vi "Tank Controll.vi"() -> ()   [LabVIEW 2016]
uses:
  <vilib>/addons/control/pid/pid.llb/PID (DBL).vi
  <vilib>/addons/control/pid/NI_PID_pid.lvlib
  <vilib>/measure/NI_MABase.lvlib
panel:
  out "String 2":string
  out "String":string
  in  "Cycle Stop":bool
  in  "Start":bool
  in  "Position 2":bool
  in  "Position 1":bool
  out "Conveyor":bool
  out "Drop 2":bool
  out "Drop 1":bool
  out "Fill Two":bool
  out "Fill One":bool
  in  "Tank Controll":bool
  in  "Setpoint  2":dbl
  in  "level 2":dbl(slide) scale=0.0..10.0
  out "Pump on":bool
  in  "Setpoint":dbl
  in  "stop":bool
  in  "level":dbl(slide) scale=0.0..10.0
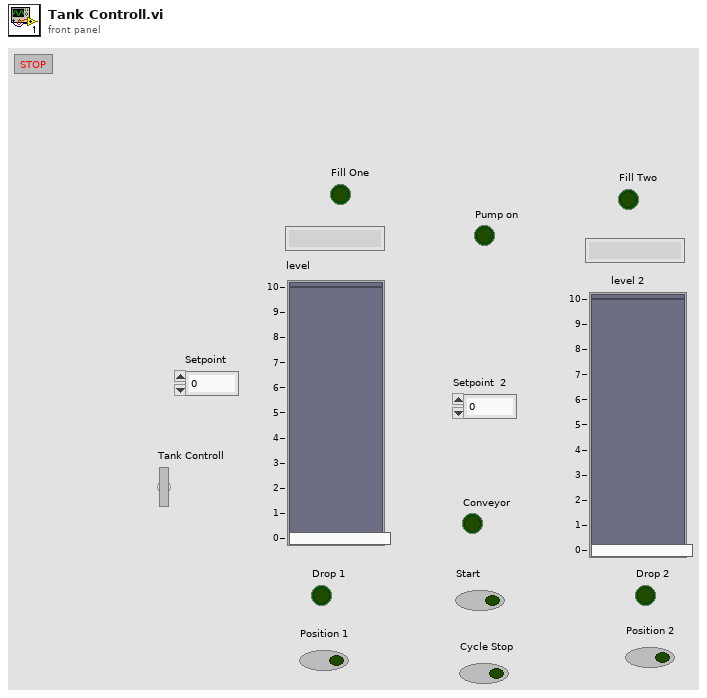
[diagram p1: front panel]
types:
  T1 = enum16{"Wait For Start", "Move Tank 1", "Fill One", "Move Tank 2", "Fill Two", "Move to Stop", "Stop All"}
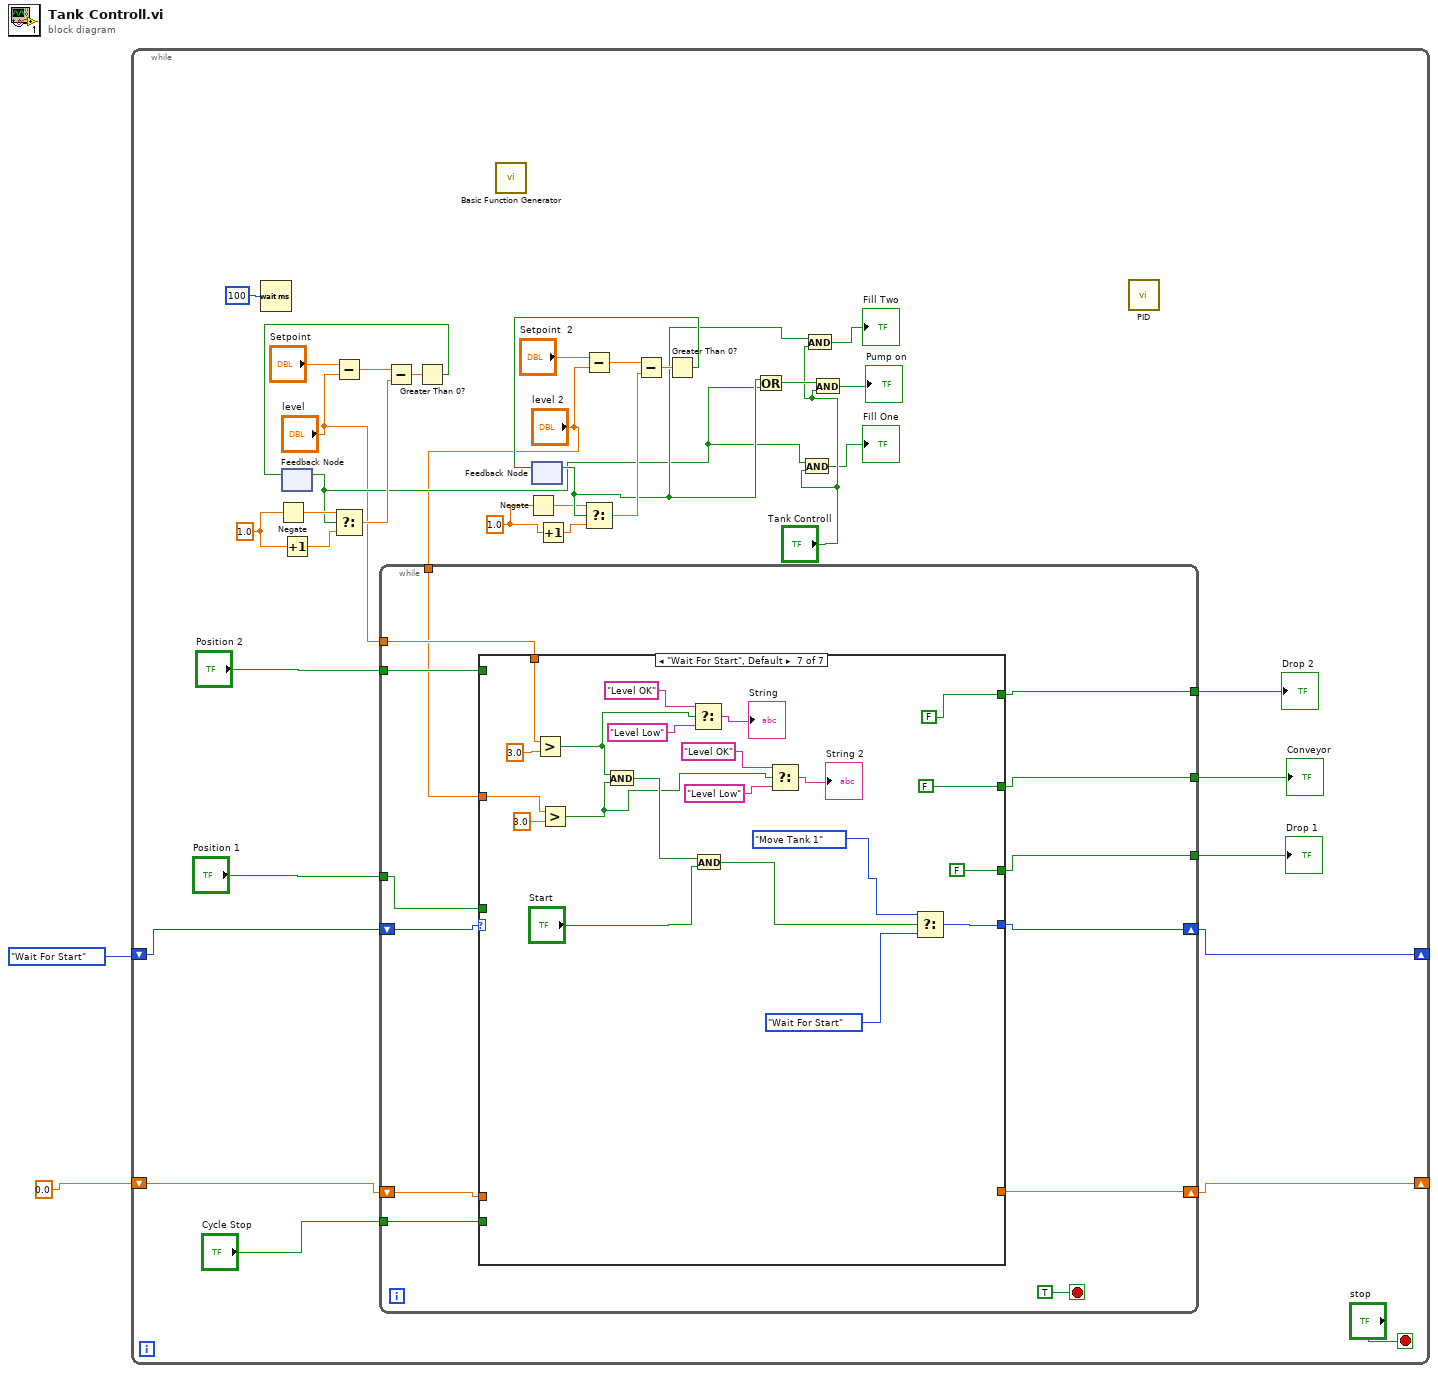
[diagram p0: block diagram]
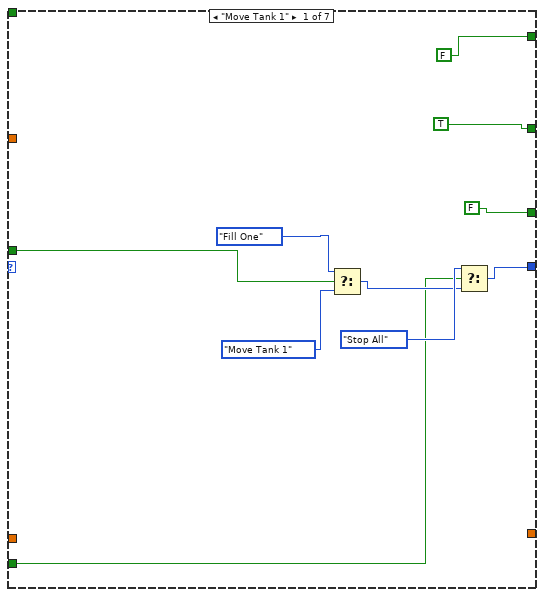
[diagram p2: hidden frame]
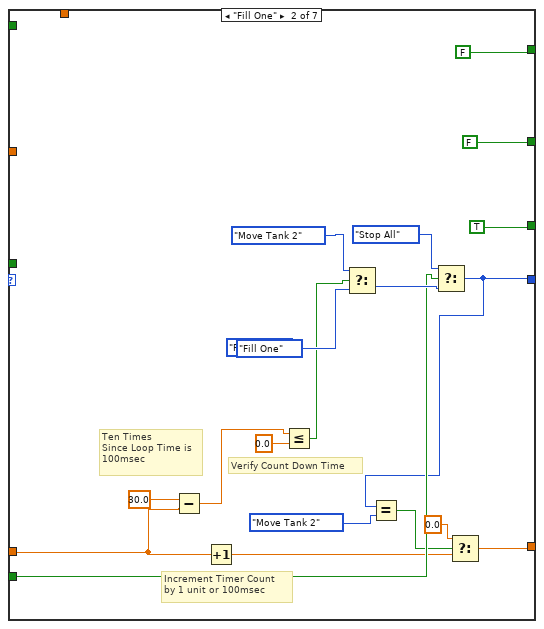
[diagram p3: hidden frame]
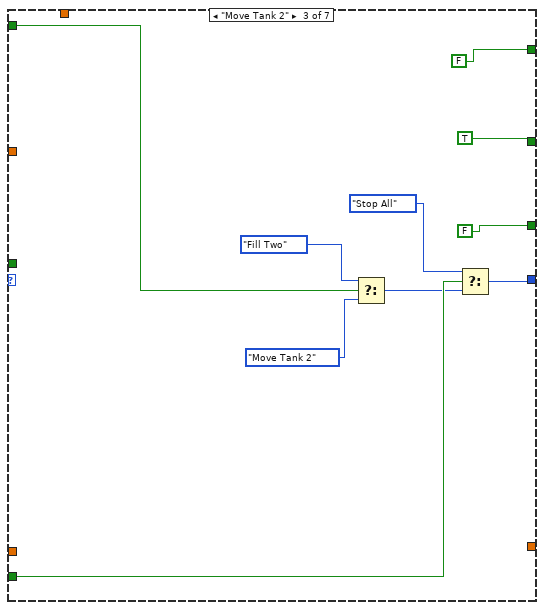
[diagram p4: hidden frame]
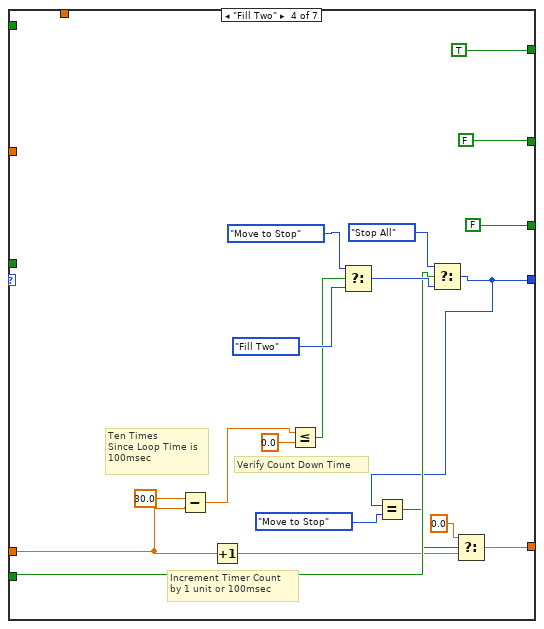
[diagram p5: hidden frame]
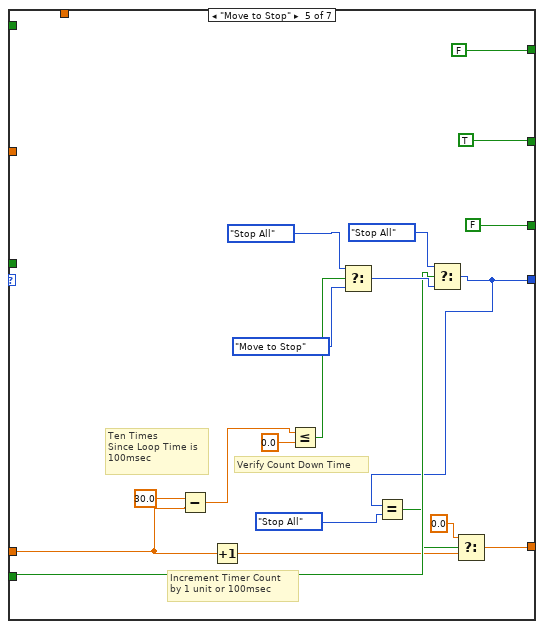
[diagram p6: hidden frame]
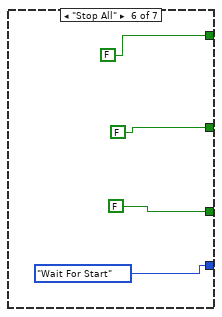
[diagram p7: hidden frame]
diagram:
  n1 = while {
    shift-right: [w13] -> _
    shift-left: T1."Wait For Start" -> [w14]
    shift-right: [w10] -> _
    shift-left: 0.0 ("Time Target (s)") -> [w11]
    stop <- "stop" stop-if-true
    w6 = 1.0 ("y")
    w9 = 1.0 ("y")
    n2 = Wait (ms)(milliseconds to wait=u32 100) -> ()  [unwired: 1 out]
    n3 = Negate(x=w9) -> (-x=w32:dbl)
    n4 = feedback #1() -> (w22:bool)  [unwired: 1 in]
    n5 = Increment(x=w9) -> (x+1=w8:dbl)
    n6 = Subtract(x="Setpoint", y="level") -> (x-y=w35:dbl)
    n7 = Select(t=w32, s=w22, f=w8) -> (s? t:f=w37:dbl)
    n8 = while {
      tunnel: "Position 2" -> [w45]
      tunnel: "Position 1" -> [w49]
      shift-right: [w51] -> w13
      shift-left: w14 -> [w50]
      tunnel: [w48] -> w17
      tunnel: [w47] -> w16
      tunnel: [w46] -> w15
      tunnel: "Cycle Stop" -> [w44]
      shift-right: [w42] -> w10
      shift-left: w11 -> [w43]
      tunnel: "level" -> [w41]
      tunnel: "level 2" -> [w40]
      stop <- TRUE stop-if-true
      n9 = case shown="\"Wait For Start\", Default" w50 {
        tunnel: [w54 w63 w82 w93 w112 T1."Wait For Start" w152] -> w51
        tunnel: [FALSE ("Drop 2") FALSE ("Drop 2") FALSE ("Drop 2") TRUE ("Drop 2") FALSE ("Drop 2") FALSE ("Drop 2") FALSE ("Drop 2")] -> w48
        tunnel: [TRUE ("Drop 2") FALSE ("Drop 2") TRUE ("Drop 2") FALSE ("Drop 2") TRUE ("Drop 2") FALSE ("Drop 2") FALSE ("Drop 2")] -> w47
        tunnel: [FALSE ("Drop 2") TRUE ("Drop 2") FALSE ("Drop 2") FALSE ("Drop 2") FALSE ("Drop 2") FALSE ("Drop 2") FALSE ("Drop 2")] -> w46
        tunnel: w49 -> [w57 _ _ _ _ _ _]
        tunnel: w45 -> [_ _ w86 _ _ _ _]
        tunnel: w44 -> [w53 w74 w85 w106 w125 _ _]
        tunnel: w43 -> [_ w65 _ w96 w115 _ _]
        tunnel: [_ w66 _ w92 w111 _ _] -> w42
        tunnel: w41 -> [_ _ _ _ _ _ w143]
        tunnel: w40 -> [_ _ _ _ _ _ w142]
        frame "Move Tank 1" {
          n10 = Select(t=T1."Fill One", s=w57, f=T1."Move Tank 1") -> (s? t:f=w55:T1)
          n11 = Select(t=T1."Stop All", s=w53, f=w55) -> (s? t:f=w54:T1)
        }
        frame "Fill One" {
          (unwired) T1."Fill One"
          # "Increment Timer Count \nby 1 unit or 100msec"
          # "Verify Count Down Time"
          # "Ten Times\nSince Loop Time is\n100msec"
          n12 = Subtract(x=30.0, y=w65) -> (x-y=w73:dbl)
          n13 = Increment(x=w65) -> (x+1=w69:dbl)
          n14 = Less Or Equal?(x=w73, y=0.0) -> (x <= y?=w64:bool)
          n15 = Select(t=T1."Move Tank 2", s=w64, f=T1."Fill One") -> (s? t:f=w76:T1)
          n16 = Select(t=T1."Stop All", s=w74, f=w76) -> (s? t:f=w63:T1)
          n17 = Equal?(x=w63, y=T1."Move Tank 2") -> (x = y?=w70:bool)
          n18 = Select(t=0.0 ("y"), s=w70, f=w69) -> (s? t:f=w66:dbl)
        }
        frame "Move Tank 2" {
          n19 = Select(t=T1."Fill Two", s=w86, f=T1."Move Tank 2") -> (s? t:f=w83:T1)
          n20 = Select(t=T1."Stop All", s=w85, f=w83) -> (s? t:f=w82:T1)
        }
        frame "Fill Two" {
          # "Increment Timer Count \nby 1 unit or 100msec"
          # "Verify Count Down Time"
          # "Ten Times\nSince Loop Time is\n100msec"
          n21 = Subtract(x=30.0, y=w96) -> (x-y=w102:dbl)
          n22 = Increment(x=w96) -> (x+1=w98:dbl)
          n23 = Less Or Equal?(x=w102, y=0.0) -> (x <= y?=w94:bool)
          n24 = Select(t=T1."Move to Stop", s=w94, f=T1."Fill Two") -> (s? t:f=w109:T1)
          n25 = Select(t=T1."Stop All", s=w106, f=w109) -> (s? t:f=w93:T1)
          n26 = Equal?(x=w93, y=T1."Move to Stop") -> (x = y?=w99:bool)
          n27 = Select(t=0.0 ("y"), s=w99, f=w98) -> (s? t:f=w92:dbl)
        }
        frame "Move to Stop" {
          # "Increment Timer Count \nby 1 unit or 100msec"
          # "Verify Count Down Time"
          # "Ten Times\nSince Loop Time is\n100msec"
          n28 = Subtract(x=30.0, y=w115) -> (x-y=w121:dbl)
          n29 = Increment(x=w115) -> (x+1=w117:dbl)
          n30 = Less Or Equal?(x=w121, y=0.0) -> (x <= y?=w113:bool)
          n31 = Select(t=T1."Stop All", s=w113, f=T1."Move to Stop") -> (s? t:f=w128:T1)
          n32 = Select(t=T1."Stop All", s=w125, f=w128) -> (s? t:f=w112:T1)
          n33 = Equal?(x=w112, y=T1."Stop All") -> (x = y?=w118:bool)
          n34 = Select(t=0.0 ("y"), s=w118, f=w117) -> (s? t:f=w111:dbl)
        }
        frame "Stop All" {
        }
        frame "Wait For Start", Default {
          n35 = Greater?(x=w143, y=3.0) -> (0:w139:bool)
          n36 = Greater?(x=w142, y=3.0) -> (0:w134:bool)
          n37 = And(x=w139, y=w134) -> (x .and. y?=w146:bool)
          n38 = Select(t="Level OK", s=w139, f="Level Low") -> (s? t:f=→"String":string)
          n39 = And(x=w146, y="Start") -> (x .and. y?=w144:bool)
          n40 = Select(t="Level OK", s=w134, f="Level Low") -> (s? t:f=→"String 2":string)
          n41 = Select(t=T1."Move Tank 1", s=w144, f=T1."Wait For Start") -> (s? t:f=w152:T1)
        }
      }
    }
    "Drop 2" <- w17
    "Conveyor" <- w16
    "Drop 1" <- w15
    n42 = Subtract(x=w35, y=w37) -> (x-y=w38:dbl)
    n43 = Greater Than 0?(x=w38) -> (x > 0?=w34:bool)
    n44 = feedback-in #1(w34) -> ()
    n45 = call <vilib>:"Basic Function Generator.vi"() -> ()  [unwired: 9 in, 3 out]
    n46 = Negate(x=w6) -> (-x=w7:dbl)
    n47 = feedback #2() -> (w24:bool)  [unwired: 1 in]
    n48 = Increment(x=w6) -> (x+1=w5:dbl)
    n49 = Subtract(x="Setpoint  2", y="level 2") -> (x-y=w28:dbl)
    n50 = Select(t=w7, s=w24, f=w5) -> (s? t:f=w30:dbl)
    n51 = Subtract(x=w28, y=w30) -> (x-y=w31:dbl)
    n52 = Greater Than 0?(x=w31) -> (x > 0?=w27:bool)
    n53 = feedback-in #2(w27) -> ()
    n54 = Or(x=w24, y=w22) -> (x .or. y?=w26:bool)
    n55 = And(x=w22, y="Tank Controll") -> (x .and. y?=→"Fill One":bool)
    n56 = And(x=w24, y="Tank Controll") -> (x .and. y?=→"Fill Two":bool)
    n57 = And(x=w26, y="Tank Controll") -> (x .and. y?=→"Pump on":bool)
    n58 = call-poly <vilib>:"PID.vi"() -> ()  [unwired: 10 in, 2 out]
  }
